vi "arduinotanque.vi"() -> ()   [LabVIEW 2013]
uses:
  <vilib>/LabVIEW Interface for Arduino/Type Defs/Board Type.ctl
  <vilib>/LabVIEW Interface for Arduino/Type Defs/Connection Type.ctl
  <vilib>/LabVIEW Interface for Arduino/LabVIEW Interface for Arduino.lvlib
panel:
  in  "Digital I/O Pin (0) 2":u8
  in  "Digital I/O Pin (0)":u8
  in  "Connection Type (USB/Serial)":T1
  in  "Board Type (Uno)":T2
  in  "Baud Rate (115200)":u32=115200
  in  "VISA resource":refnum<visa-resource-name>
  out "Tank":dbl(slide) scale=0.0..500.0
  in  "Analog Input Pin (0)":u8
  in  "stop":bool
  # "UNIVERSIDAD DE CUNDINAMARCA\nINGENIERIA DE SISTEMAS\nELECTIVA PROFESIONAL IV\nANDY CAMARGO\nRAFAEL REYES\nSEMESTRE X\nEXTENCION CHIA"
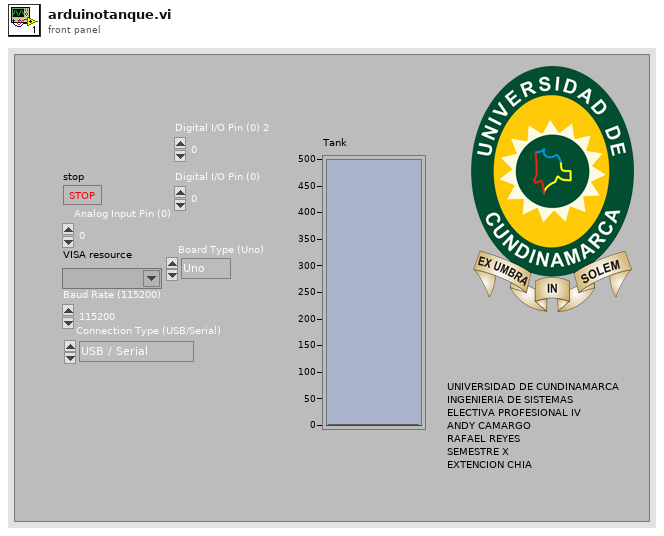
[diagram p1: front panel]
types:
  T1 = typedef "LabVIEW Interface for Arduino.lvlib/Connection Type.ctl" = enum8{"USB / Serial", "XBEE", "BlueSmirf (Bluetooth)"}
  T2 = typedef "LabVIEW Interface for Arduino.lvlib/Board Type.ctl" = enum16{"Uno", "Dimuelanove w/Atmega 328", "Mega 2560"}
  T3 = typedef "LabVIEW Interface for Arduino.lvlib/Arduino Resource.ctl" = cluster{"VISA resource":refnum<visa-resource-name>, "Board Type":T2, "Connection Type":enum8{"USB / Serial"}, "Bytes Per Packet (15)":u8}
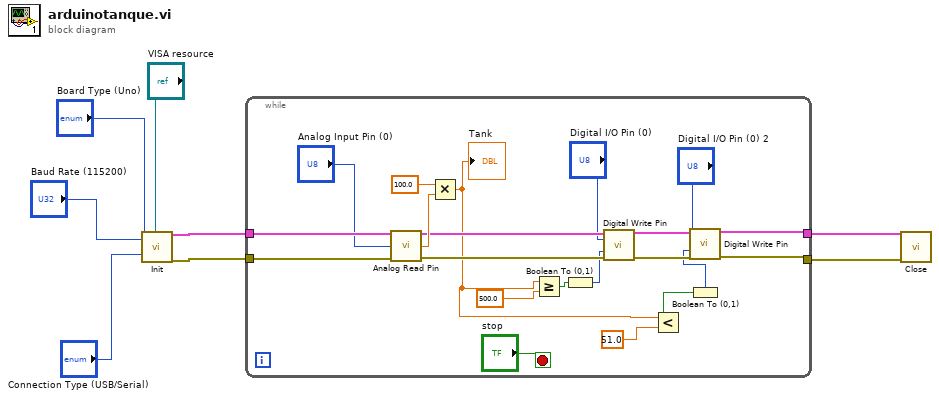
[diagram p0: block diagram]
diagram:
  n1 = call <vilib>:"Init.vi"("VISA resource"="VISA resource", "Baud Rate (115200)"="Baud Rate (115200)", "Board Type (Uno)"="Board Type (Uno)", "Connection Type (USB/Serial)"="Connection Type (USB/Serial)") -> ("Arduino Resource"=w8:T3, "error out"=w6:errorcluster)  [unwired: 14 in]
  n2 = while {
    tunnel: w8 -> [w28]
    tunnel: [w16] -> w7
    tunnel: w6 -> [w27]
    tunnel: [w14] -> w1
    stop <- "stop" stop-if-true
    n3 = call <vilib>:"Analog Read Pin.vi"("Arduino Resource"=w28, "Analog Input Pin (0)"="Analog Input Pin (0)", "error in"=w27) -> ("Arduino Resource"=w23:T3, "Voltage"=w25:dbl, "error out"=w22:errorcluster)  [unwired: 10 in]
    n4 = Multiply(x=100.0, y=w25) -> (x*y=w9:dbl)
    "Tank" <- w9
    n5 = Greater Or Equal?(x=w9, y=500.0) -> (x >= y?=w19:bool)
    n6 = Boolean To (0,1)(Boolean=w19) -> (0, 1=w20:i16)
    n7 = call <vilib>:"Digital Write Pin.vi"("Arduino Resource"=w23, "Digital I/O Pin (0)"="Digital I/O Pin (0)", "Value (0)"=w20, "error in"=w22) -> ("Arduino Resource"=w17:T3, "error out"=w15:errorcluster)  [unwired: 10 in]
    n8 = Less?(x=w9, y=51.0) -> (x < y?=w12:bool)
    n9 = Boolean To (0,1)(Boolean=w12) -> (0, 1=w11:i16)
    n10 = call <vilib>:"Digital Write Pin.vi"("Arduino Resource"=w17, "Digital I/O Pin (0)"="Digital I/O Pin (0) 2", "Value (0)"=w11, "error in"=w15) -> ("Arduino Resource"=w16:T3, "error out"=w14:errorcluster)  [unwired: 10 in]
  }
  n11 = call <vilib>:"Close.vi"("Arduino Resource"=w7, "error in"=w1) -> ()  [unwired: 13 in, 1 out]
